vi "GetLargest1DFrom2D.vi"(2 "Col No.":i32, 3 "2D Input":dbl[][](array[numeric])) -> (0 "1D Output":dbl[](array[numeric]), 1 "max index(es)":i32)   [LabVIEW 2015]
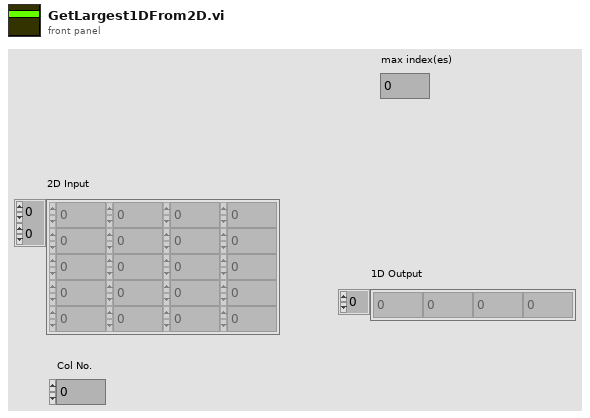
[diagram p1: front panel]
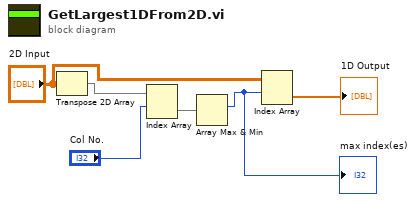
[diagram p0: block diagram]
diagram:
  n1 = Transpose 2D Array(2D array="2D Input") -> (transposed array=w4:dbl[][])
  n2 = Index Array(array=w4, index (row)="Col No.") -> (element=w5:dbl[])  [unwired: 1 in]
  n3 = Array Max & Min(array=w5) -> (max index (indices)=w3:i32)  [unwired: 3 out]
  "max index(es)" <- w3
  n4 = Index Array(array="2D Input", index (row)=w3) -> (element=→"1D Output":dbl[])  [unwired: 1 in]
